vi "binary_reader.vi"(7 "error in":errorcluster, 9 "are calibration coefficients\n available in the binary file?":bool, 10 "path to binary file":path) -> (0 "error out":errorcluster, 1 "time informations":T6 {"length" format="%<%H:%M:%S%3u>t"}, 3 "all in one package":T3={"memory structure"={"length of metadata [byte]"=5, "length of page [byte]"=2048, "length of measurement data on page [byte]"=2028, "length of dataset [byte]"=6}, "actigraph settings"={"sampling frequency [Hz]"=0.0, "measurement interval [± g]"=0, "high precision?"=FALSE, "number of pages"=0, "rate code"=0, "range code"=0, "id"=0}, "time informations"={"starting time"=timestamp(0 s since 1904-01-01), "ending time"=timestamp(0 s since 1904-01-01), "dt[s]"=0.0, "sampling rate [Hz]"=0.0, "length"=0.0}, "measurement data"={"number of samples per axis"=0, "timestamp array"=[], "offset array"=[], "x, y, z axis data"=[], "normalised magnitude of acceleartion vectors"={"t0"=timestamp(0 s since 1904-01-01), "dt"=1.0, "Y"=[]}, "calibration coefficients"={"Sx"=0.0, "Ox"=0.0, "Sy"=0.0, "Oy"=0.0, "Sz"=0.0, "Oz"=0.0}, "statistics"={"mean of x axis acceleration"=0.0, "standard devation of x axis acceleration"=0.0, "mean of y axis acceleration"=0.0, "standard devation of y axis acceleration"=0.0, "mean of z axis acceleration"=0.0, "standard devation of z axis acceleration"=0.0, "mean of normalised magnitude of acceleration"=0.0, "standard devation of normalised magnitude of acceleration"=0.0}, "battery voltage"={"t0"=timestamp(0 s since 1904-01-01), "dt"=1.0, "Y"=[]}, "magnitude of acceleartion vectors"={"t0"=timestamp(0 s since 1904-01-01), "dt"=1.0, "Y"=[]}}} {"measurement data"."calibration coefficients"."Oz" format="%#_12g"; "measurement data"."calibration coefficients"."Sz" format="%#_12g"; "measurement data"."calibration coefficients"."Oy" format="%#_12g"; "measurement data"."calibration coefficients"."Sy" format="%#_12g"; "measurement data"."calibration coefficients"."Ox" format="%#_12g"; "measurement data"."calibration coefficients"."Sx" format="%#_12g"; "time informations"."length" format="%<%H:%M:%S%3u>t"; "actigraph settings"."id" format="%02d"; "actigraph settings"."range code" format="%02x"; "actigraph settings"."rate code" format="%02x"})   [LabVIEW 2019]
uses:
  Controls/control_memory_structure.ctl
  Controls/control_time_informations.ctl
  Controls/control_measurement_settings.ctl
  Controls/control_all_in_one_package.ctl
  Controls/control_measurement_data.ctl
  Controls/control_calibration_coefficients.ctl
  Controls/control_statistics.ctl
panel:
  out "battery voltage over time":waveform(dbl)(graph)
  out "statistics":T1
  out "calibration coefficients":T2 {"Oz" format="%#_12g"; "Sz" format="%#_12g"; "Oy" format="%#_12g"; "Sy" format="%#_12g"; "Ox" format="%#_12g"; "Sx" format="%#_12g"}
  out "normalised magnitude of acceleration vectors over time":waveform(dbl)(graph)
  out "actigraph settings":T5={"sampling frequency [Hz]"=9.980607627666451, "measurement interval [± g]"=0, "high precision?"=FALSE, "number of pages"=0, "rate code"=0, "range code"=0, "id"=0} {"id" format="%02d"; "range code" format="%02x"; "rate code" format="%02x"}
  in  "memory structure":T4={"length of metadata [byte]"=5, "length of page [byte]"=2048, "length of measurement data on page [byte]"=2028, "length of dataset [byte]"=6}
  out "3 axis acceleration over time":waveform(dbl)[](graph)
  # "if this button is true, the calibration of \nacceleration vectors components are made automatically"
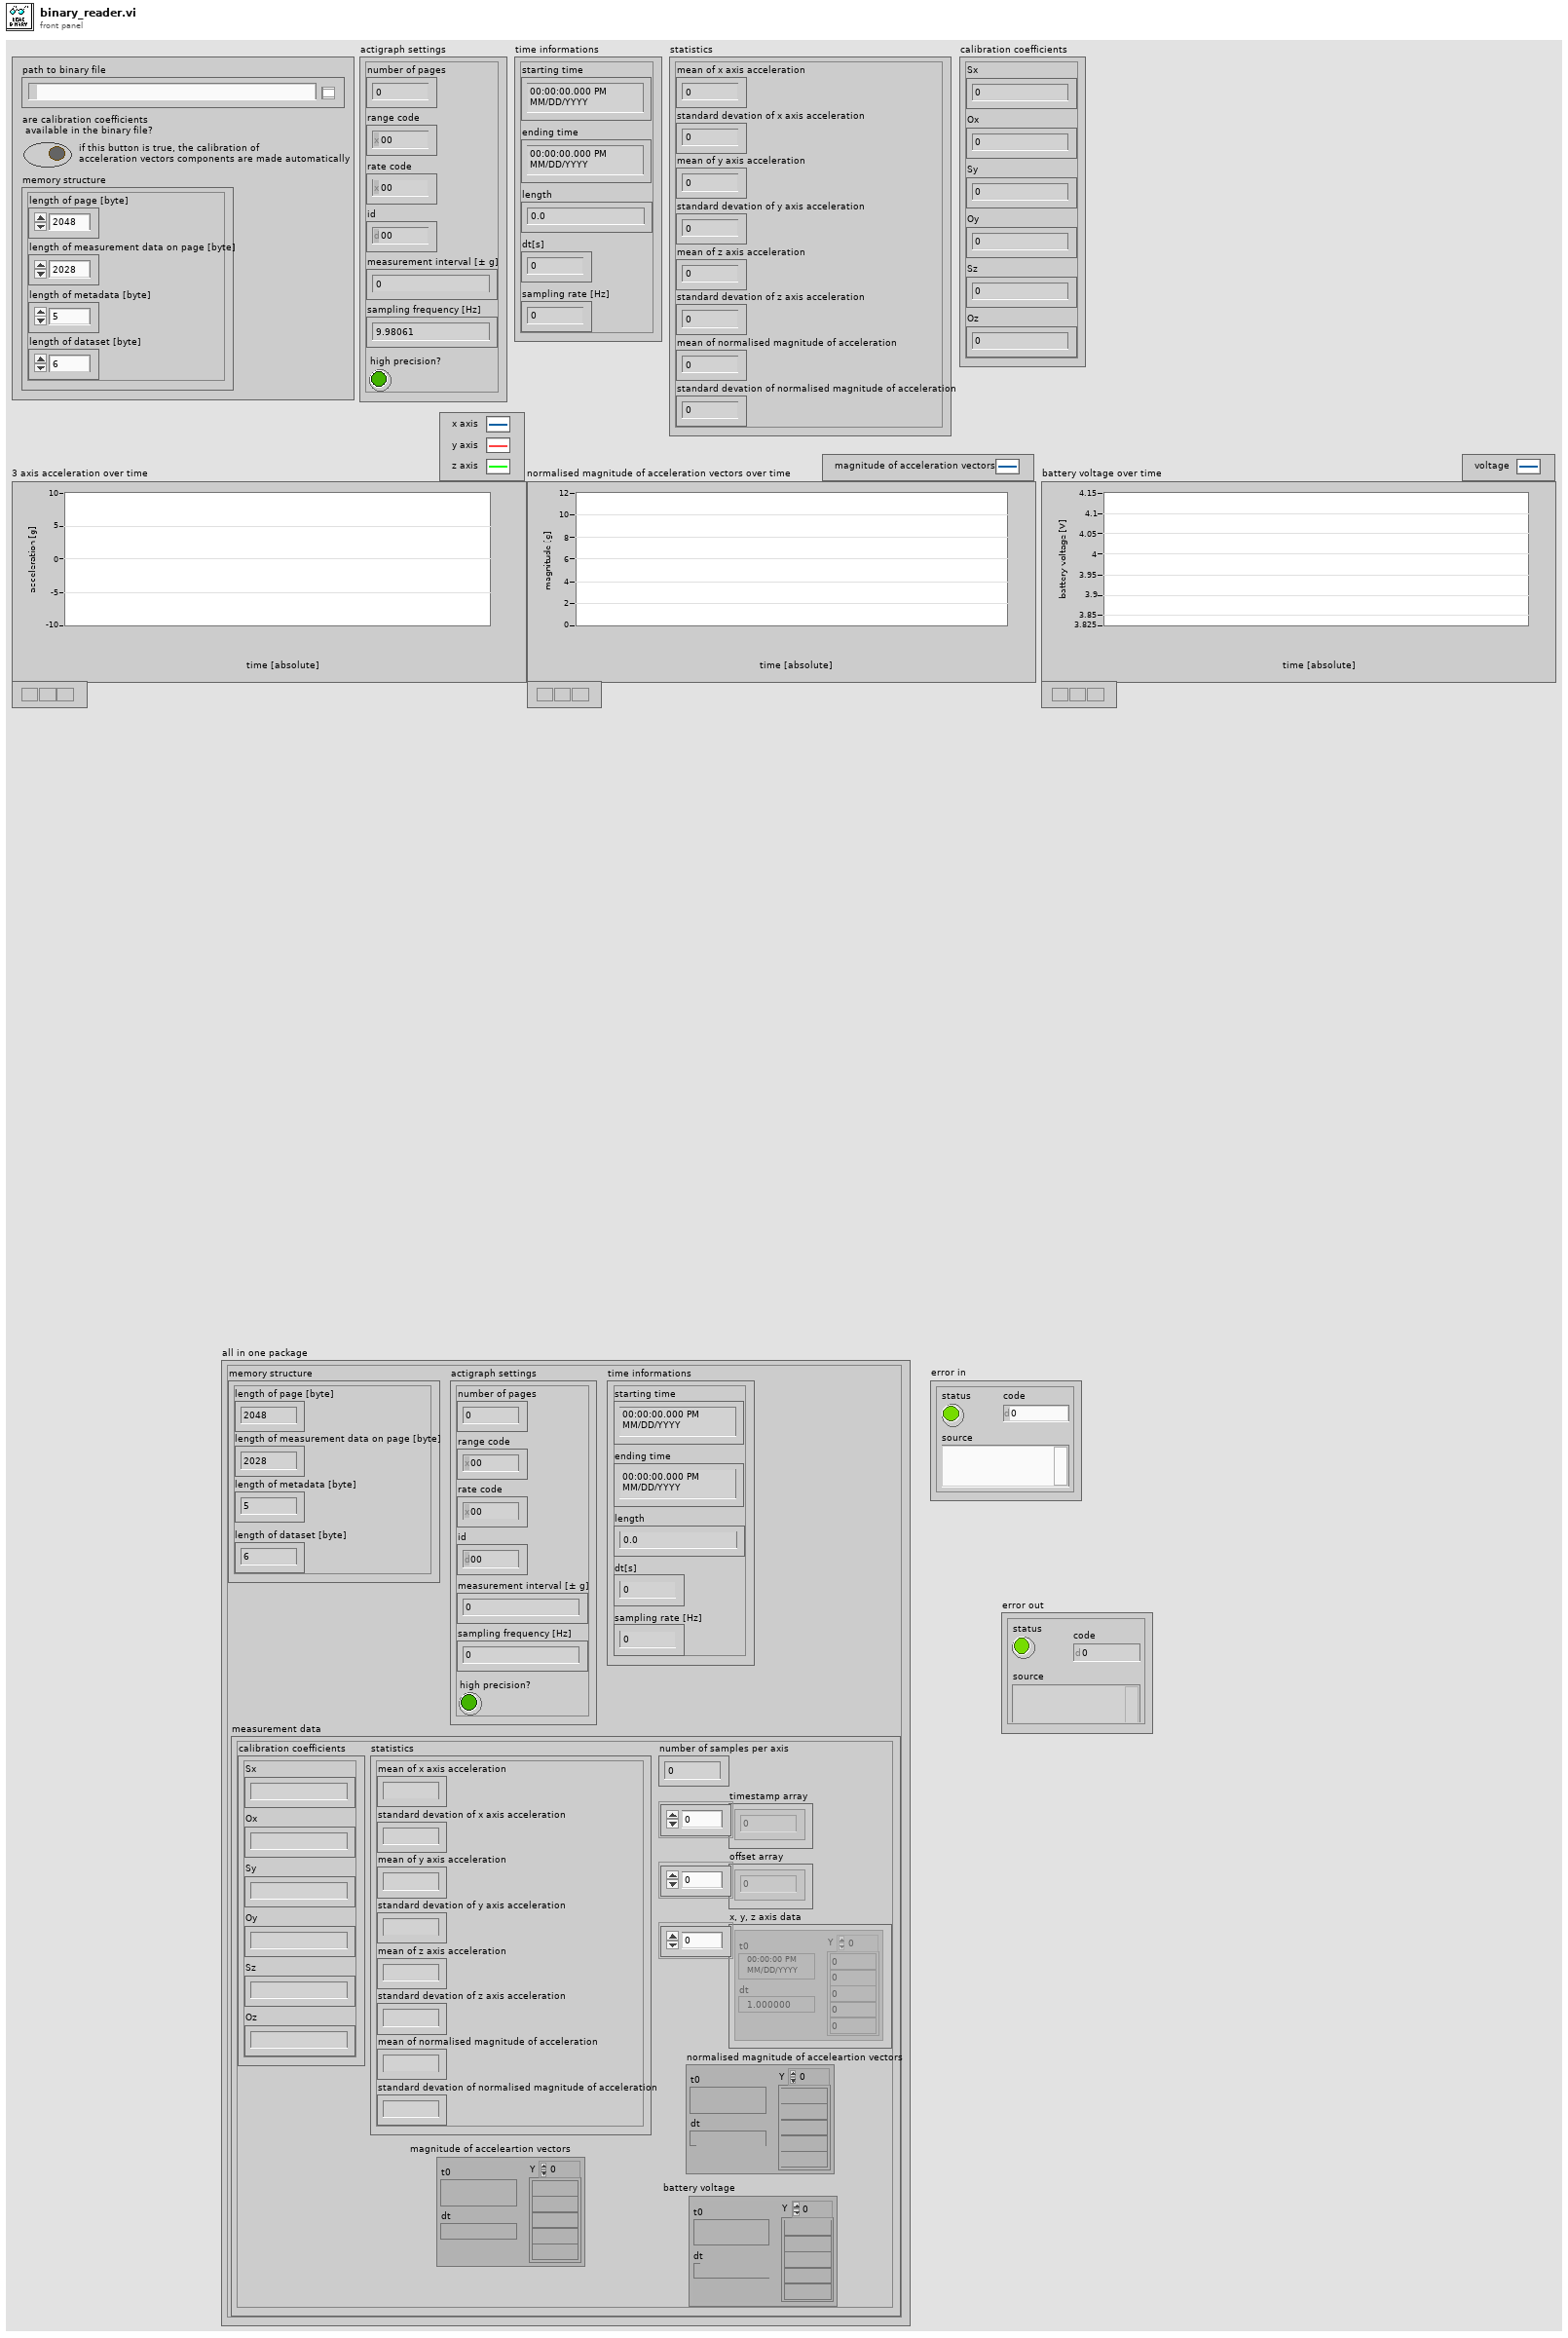
[diagram p1: front panel]
types:
  T1 = typedef "control_statistics.ctl" = cluster{"mean of x axis acceleration":dbl, "standard devation of x axis acceleration":dbl, "mean of y axis acceleration":dbl, "standard devation of y axis acceleration":dbl, "mean of z axis acceleration":dbl, "standard devation of z axis acceleration":dbl, "mean of normalised magnitude of acceleration":dbl, "standard devation of normalised magnitude of acceleration":dbl}
  T2 = typedef "control_calibration_coefficients.ctl" = cluster{"Sx":dbl, "Ox":dbl, "Sy":dbl, "Oy":dbl, "Sz":dbl, "Oz":dbl}
  T3 = typedef "control_all_in_one_package.ctl" = cluster{"memory structure":T4, "actigraph settings":T5, "time informations":T6, "measurement data":T7}
  T4 = typedef "control_memory_structure.ctl" = cluster{"length of metadata [byte]":i32, "length of page [byte]":i32, "length of measurement data on page [byte]":i32, "length of dataset [byte]":i32}
  T5 = typedef "control_measurement_settings.ctl" = cluster{"sampling frequency [Hz]":dbl, "measurement interval [± g]":i32, "high precision?":bool, "number of pages":i32, "rate code":i32, "range code":i32, "id":i32}
  T6 = typedef "control_time_informations.ctl" = cluster{"starting time":timestamp, "ending time":timestamp, "dt[s]":dbl, "sampling rate [Hz]":dbl, "length":dbl}
  T7 = typedef "control_measurement_data.ctl" = cluster{"number of samples per axis":i32, "timestamp array":dbl[], "offset array":dbl[], "x, y, z axis data":waveform(dbl)[], "normalised magnitude of acceleartion vectors":waveform(dbl), "calibration coefficients":T2, "statistics":T1, "battery voltage":waveform(dbl), "magnitude of acceleartion vectors":waveform(dbl)}
  T8 = cluster{"mean of x axis acceleration":dbl, "standard devation of x axis acceleration":dbl, "mean of y axis acceleration":dbl, "standard devation of y axis acceleration":dbl, "mean of z axis acceleration":dbl, "standard devation of z axis acceleration":dbl, "mean of magnitude of acceleration":dbl, "standard devation of magnitude of acceleration":dbl}
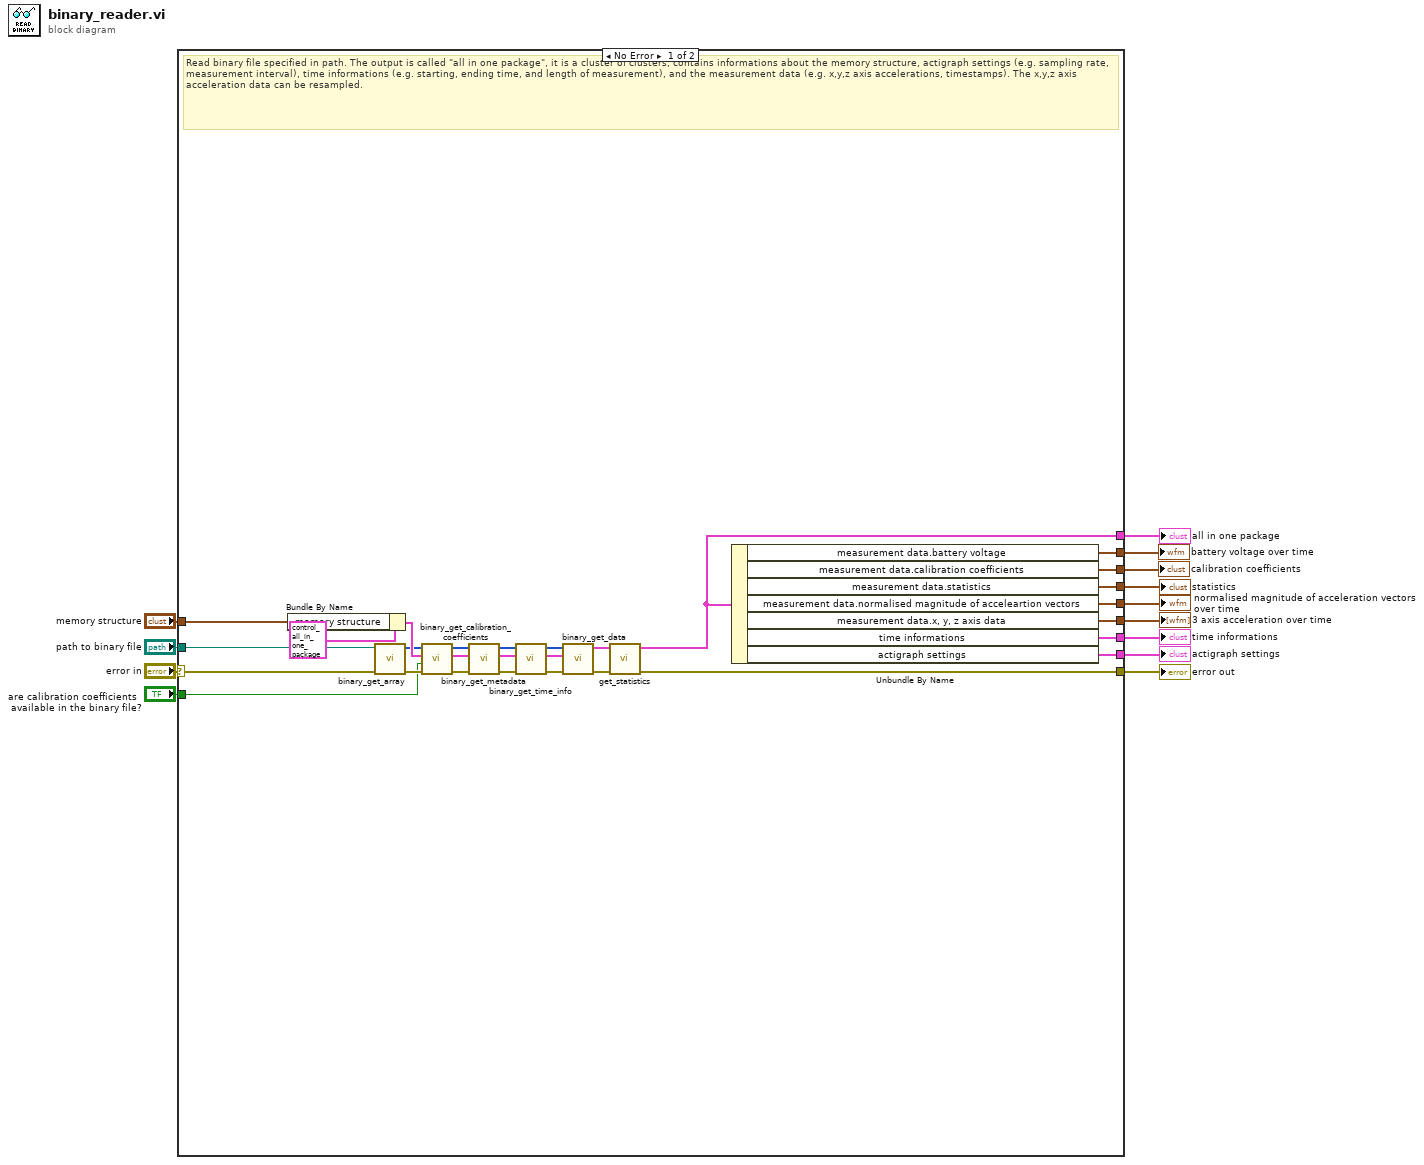
[diagram p0: block diagram]
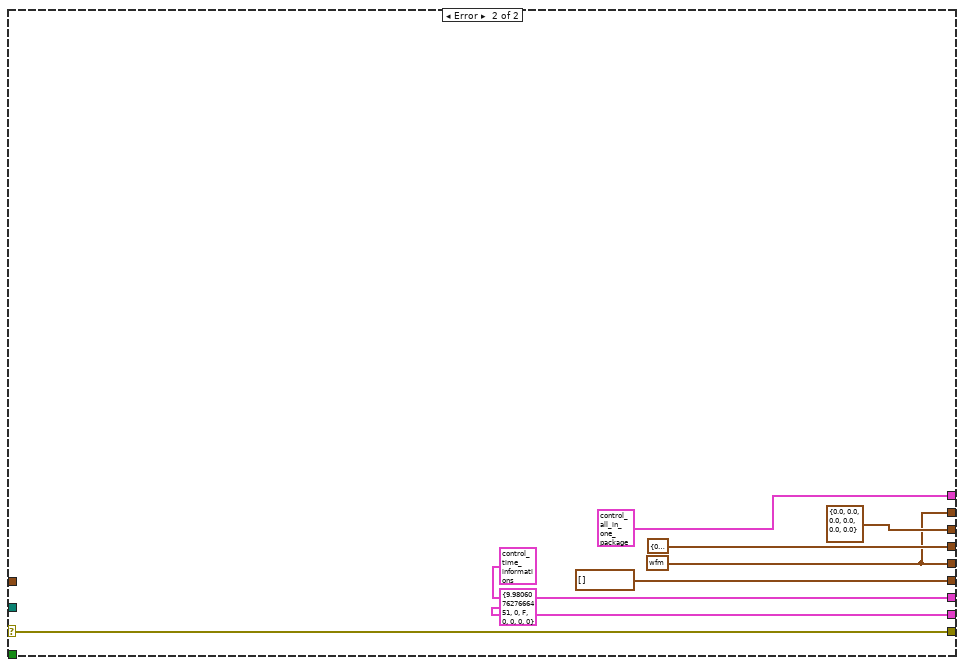
[diagram p2: hidden frame]
diagram:
  n1 = case shown="No Error" "error in" {
    selector: "error in" -> [w30 w49]
    tunnel: "path to binary file" -> [w40 _]
    tunnel: "memory structure" -> [w36 _]
    tunnel: [w27 w49] -> w12
    tunnel: [w35 waveform(dbl)[] [] ("x, y, z axis data")] -> w6
    tunnel: [w33 T6 {"starting time"=timestamp(0 s since 1904-01-01), "ending time"=timestamp(0 s since 1904-01-01), "dt[s]"=0.0, "sampling rate [Hz]"=0.0, "length"=0.0} ("time informations")] -> w8
    tunnel: [w32 T5 {"sampling frequency [Hz]"=9.980607627666451, "measurement interval [± g]"=0, "high precision?"=FALSE, "number of pages"=0, "rate code"=0, "range code"=0, "id"=0} ("actigraph settings")] -> w11
    tunnel: [w26 T3 {"memory structure"={"length of metadata [byte]"=5, "length of page [byte]"=2048, "length of measurement data on page [byte]"=2028, "length of dataset [byte]"=6}, "actigraph settings"={"sampling frequency [Hz]"=0.0, "measurement interval [± g]"=0, "high precision?"=FALSE, "number of pages"=0, "rate code"=0, "range code"=0, "id"=0}, "time informations"={"starting time"=timestamp(0 s since 1904-01-01), "ending time"=timestamp(0 s since 1904-01-01), "dt[s]"=0.0, "sampling rate [Hz]"=0.0, "length"=0.0}, "measurement data"={"number of samples per axis"=0, "timestamp array"=[], "offset array"=[], "x, y, z axis data"=[], "normalised magnitude of acceleartion vectors"={"t0"=timestamp(0 s since 1904-01-01), "dt"=1.0, "Y"=[]}, "calibration coefficients"={"Sx"=0.0, "Ox"=0.0, "Sy"=0.0, "Oy"=0.0, "Sz"=0.0, "Oz"=0.0}, "statistics"={"mean of x axis acceleration"=0.0, "standard devation of x axis acceleration"=0.0, "mean of y axis acceleration"=0.0, "standard devation of y axis acceleration"=0.0, "mean of z axis acceleration"=0.0, "standard devation of z axis acceleration"=0.0, "mean of normalised magnitude of acceleration"=0.0, "standard devation of normalised magnitude of acceleration"=0.0}, "battery voltage"={"t0"=timestamp(0 s since 1904-01-01), "dt"=1.0, "Y"=[]}, "magnitude of acceleartion vectors"={"t0"=timestamp(0 s since 1904-01-01), "dt"=1.0, "Y"=[]}}} ("all in one package out")] -> w9
    tunnel: [w29 w42] -> w5
    tunnel: [w28 T8 {"mean of x axis acceleration"=0.0, "standard devation of x axis acceleration"=0.0, "mean of y axis acceleration"=0.0, "standard devation of y axis acceleration"=0.0, "mean of z axis acceleration"=0.0, "standard devation of z axis acceleration"=0.0, "mean of magnitude of acceleration"=0.0, "standard devation of magnitude of acceleration"=0.0} ("statistics")] -> w2
    tunnel: "are calibration coefficients\n available in the binary file?" -> [w18 _]
    tunnel: [w17 T2 {"Sx"=0.0, "Ox"=0.0, "Sy"=0.0, "Oy"=0.0, "Sz"=0.0, "Oz"=0.0} ("Calibration coefficients")] -> w3
    tunnel: [w16 w42] -> w1
    frame No Error {
      # "Read binary file specified in path. The output is called \"all in one package\", it is a cluster of clusters, contains informations about the memory structure, actigraph settings (e.g. sampling rate, measurement interval), time informations (e.g. starting, ending time, and length of measurement), and the measurement data (e.g. x,y,z axis accelerations, timestamps). The x,y,z axis acceleration data can be resampled."
      n2 = Bundle By Name(cluster=T3 {"memory structure"={"length of metadata [byte]"=5, "length of page [byte]"=2048, "length of measurement data on page [byte]"=2028, "length of dataset [byte]"=6}, "actigraph settings"={"sampling frequency [Hz]"=0.0, "measurement interval [± g]"=0, "high precision?"=FALSE, "number of pages"=0, "rate code"=0, "range code"=0, "id"=0}, "time informations"={"starting time"=timestamp(0 s since 1904-01-01), "ending time"=timestamp(0 s since 1904-01-01), "dt[s]"=0.0, "sampling rate [Hz]"=0.0, "length"=0.0}, "measurement data"={"number of samples per axis"=0, "timestamp array"=[], "offset array"=[], "x, y, z axis data"=[], "normalised magnitude of acceleartion vectors"={"t0"=timestamp(0 s since 1904-01-01), "dt"=1.0, "Y"=[]}, "calibration coefficients"={"Sx"=0.0, "Ox"=0.0, "Sy"=0.0, "Oy"=0.0, "Sz"=0.0, "Oz"=0.0}, "statistics"={"mean of x axis acceleration"=0.0, "standard devation of x axis acceleration"=0.0, "mean of y axis acceleration"=0.0, "standard devation of y axis acceleration"=0.0, "mean of z axis acceleration"=0.0, "standard devation of z axis acceleration"=0.0, "mean of normalised magnitude of acceleration"=0.0, "standard devation of normalised magnitude of acceleration"=0.0}, "battery voltage"={"t0"=timestamp(0 s since 1904-01-01), "dt"=1.0, "Y"=[]}, "magnitude of acceleartion vectors"={"t0"=timestamp(0 s since 1904-01-01), "dt"=1.0, "Y"=[]}}} ("all in one package"), "memory structure"=w36) -> (w22:T3)
      n3 = call "binary_get_array.vi"("error in"=w30, "path to binary file"=w40) -> ("error out"=w23:errorcluster, "binary data"=w21:u8[])  [unwired: 8 in]
      n4 = call "binary_get_calibration_coefficients.vi"("error in"=w23, "calibrations?"=w18, "all in one package input"=w22, "binary data"=w21) -> ("error out"=w24:errorcluster, "all in one package output"=w19:T3, "binary data w/ calibration coefficients"=w20:u8[])  [unwired: 5 in]
      n5 = call "binary_get_metadata.vi"("error in"=w24, "all in one package in"=w19, "binary data w/ calibration coefficients"=w20) -> ("error out"=w41:errorcluster, "all in one package out"=w34:T3, "pages"=w39:u8[])  [unwired: 6 in]
      n6 = call "binary_get_time_info.vi"("error in"=w41, "all in one package in"=w34, "pages"=w39) -> ("error out"=w38:errorcluster, "all in one package out"=w31:T3, "pages w/ first and last page"=w37:u8[])  [unwired: 6 in]
      n7 = call "binary_get_data.vi"("error in"=w38, "all in one package in"=w31, "pages w/ first and last page"=w37) -> ("error out"=w14:errorcluster, "all in one package out"=w15:T3)  [unwired: 7 in]
      n8 = call "get_statistics.vi"("error in"=w14, "all in one package in"=w15) -> ("error out"=w27:errorcluster, "all in one package out"=w26:T3)  [unwired: 8 in]
      n9 = Unbundle By Name(w26) -> ("measurement data.battery voltage"=w16:waveform(dbl), "measurement data.calibration coefficients"=w17:T2, "measurement data.statistics"=w28:T1, "measurement data.normalised magnitude of acceleartion vectors"=w29:waveform(dbl), "measurement data.x, y, z axis data"=w35:waveform(dbl)[], "time informations"=w33:T6, "actigraph settings"=w32:T5)
    }
    frame Error {
      w42 = waveform(dbl) {"t0"=timestamp(0 s since 1904-01-01), "dt"=1.0, "Y"=[]} ("magnitude of acceleartion vectors")
    }
  }
  "error out" <- w12
  "3 axis acceleration over time" <- w6
  "time informations" <- w8
  "actigraph settings" <- w11
  "all in one package" <- w9
  "normalised magnitude of acceleration vectors over time" <- w5
  "calibration coefficients" <- w3
  "statistics" <- w2
  "battery voltage over time" <- w1
